vi "Get Channel Properties.vi"(7 "TypeName":string, 8 "error in":errorcluster, 11 "JSON":string) -> (0 "error out":errorcluster, 3 "Channel Properties":variant)   [LabVIEW 2026, in "Template Deployment Hooks.lvlib"]
uses:
  Template Deployment Hooks.lvlib
  19d9522f-46a0-4adf-8cfc-289ca929d126.vi
  <vilib>/JDP Science/JSONtext/JSON text to Variant.vi
  <vilib>/JDP Science/JSONtext/LVClass Serializer/JSONtext LVClass Serializer.lvclass
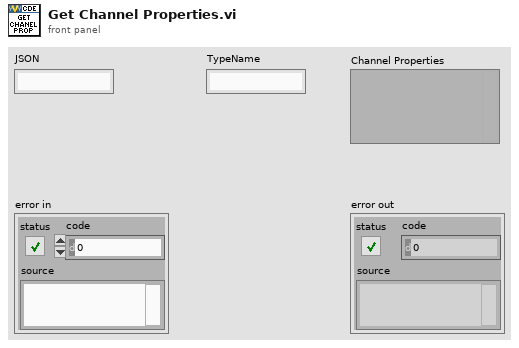
[diagram p1: front panel]
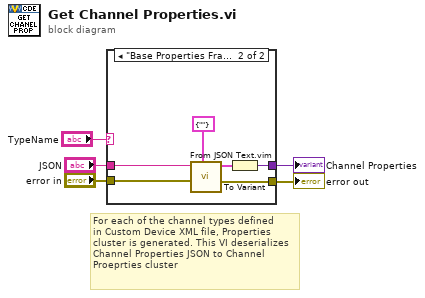
[diagram p0: block diagram]
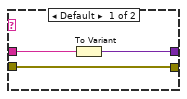
[diagram p2: hidden frame]
diagram:
  # "For each of the channel types defined\nin Custom Device XML file, Properties\ncluster is generated. This VI deserializes\nChannel Properties JSON to Channel\nProeprties cluster"
  n1 = case shown="\"Base Properties Frame\"" "TypeName" {
    tunnel: [w7 w12] -> w3
    tunnel: "error in" -> [w8 w14]
    tunnel: [w8 w13] -> w4
    tunnel: "JSON" -> [w6 w9]
    frame Default {
      n2 = To Variant(anything=w6) -> (Variant=w7:variant)
    }
    frame "Base Properties Frame" {
      n3 = call "From JSON Text.vim"("Data Type and Default Value"=cluster{string} {""} ("Properties"), "error in (no error)"=w14, "JSON"=w9) -> ("error out"=w13:errorcluster, "Data out"=w11:cluster{string})  [unwired: 7 in]
      n4 = To Variant(anything=w11) -> (Variant=w12:variant)
    }
  }
  "Channel Properties" <- w3
  "error out" <- w4
